vi "Register by Label.vi"(8 "error in (no error)":errorcluster, 9 "Observer":refnum<class "Send.lvclass">, 10 "Label to Register For":string) -> (0 "error out":errorcluster, 3 "ObserverRegistryCommand_RegisterByLabel out":refnum<class "Observer_RegisterByLabel.lvclass">)   [LabVIEW 2011, in "Messenging.lvlib" / "Observer_RegisterByLabel.lvclass"]
uses:
  Commands/Register by Label/Observer_RegisterByLabel.lvclass
  Interprocess Messenger/Send/Send.lvclass
  Commands/Register by Label/Observer_RegisterByLabel.lvclass/Observer_RegisterByLabel.ctl
  Commands/ParentCommand/ObserverRegistryCommand.lvclass
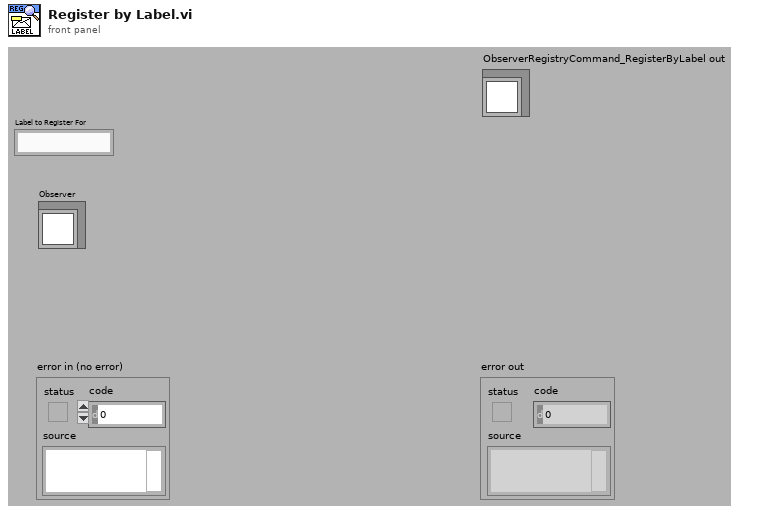
[diagram p1: front panel]
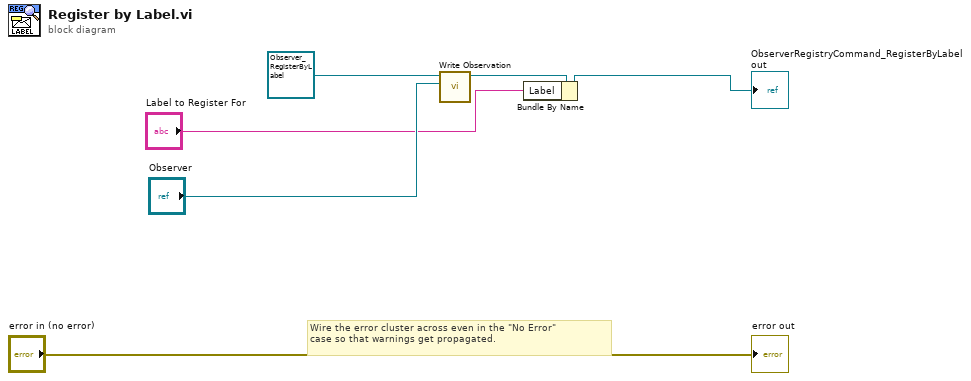
[diagram p0: block diagram]
diagram:
  # "Wire the error cluster across even in the \"No Error\"\ncase so that warnings get propagated."
  n1 = call "Write Observation.vi"("Observer"="Observer", "ObserverRegistryCommand.lvclass in"=refnum<class "Observer_RegisterByLabel.lvclass"> refnum ("ObserverRegistryCommand_RegisterByLabel in")) -> ("ObserverRegistryCommand.lvclass out"=w4:refnum<class "Observer_RegisterByLabel.lvclass">)  [unwired: 1 in, 8 out]
  n2 = Bundle By Name(cluster=w4, "Label"="Label to Register For") -> (→"ObserverRegistryCommand_RegisterByLabel out":refnum<class "Observer_RegisterByLabel.lvclass">)
  "error out" <- "error in (no error)"
